vi "testRollover.vi"() -> ()   [LabVIEW 2017]
uses:
  <vilib>/addons/InsightCM/Utilities/Analysis/Vibration/controls/digital tach state.ctl
  <vilib>/addons/InsightCM/Utilities/Analysis/Vibration/controls/tach state.ctl
  <vilib>/addons/InsightCM/Devices/Shared/VibrationAnalysisLoop/controls/TachometerChanAnalysisCfg.ctl
panel:
  out "stopped":bool
  out "Instant RPM":dbl
  out "next block":dbl[](array[numeric])
  out "x/y":dbl[](array[numeric])
  out "seconds":i32
  in  "Stop":bool
  in  "Tachometer":cluster{"RPM":sgl}={"RPM"=60.0} {"RPM" scale=1.0..6000.0}
  in  "Vibration":T1(array[cluster])
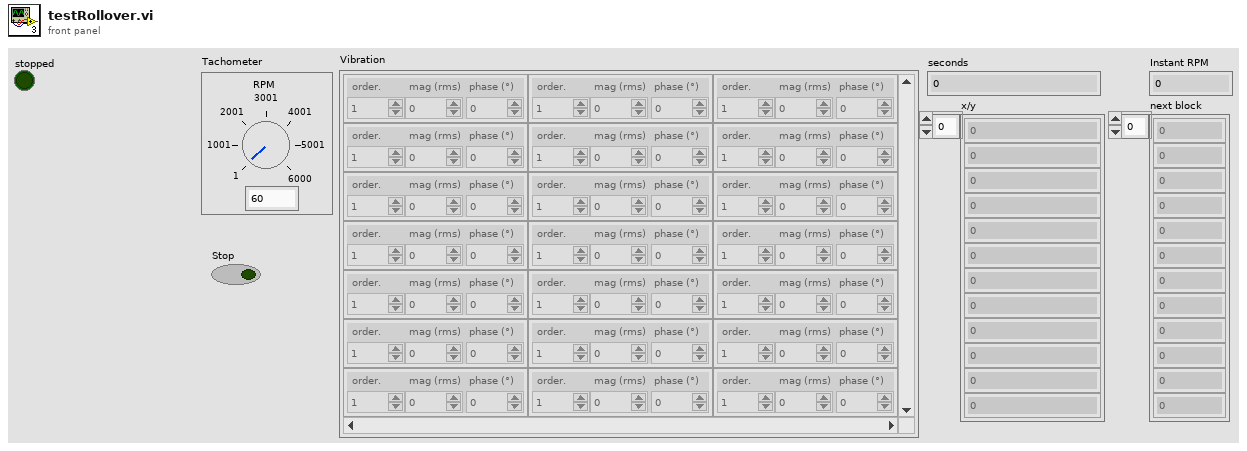
[diagram p1: front panel]
types:
  T1 = cluster{"order.":dbl, "mag (rms)":dbl, "phase (°)":dbl}[][]
  T2 = typedef "tach state.ctl" = cluster{"analog tach state":cluster{"last value":dbl, "edge state":cluster{"processed data":dbl, "buffer data":dbl[]}}, "speed state":cluster{"state":enum16{"0 Pulses", "1 Pulse", "2+ Pulses"}, "last pulse position":dbl, "RPM":dbl, "Empty Blocks":i32}, "Reset":bool, "digital tach state in":T3}
  T3 = typedef "digital tach state.ctl" = cluster{dbl[], i32, "not enough pulses?":bool, "pulse buffer out":dbl[], i32, "final state":dbl[], "duration":dbl, "reset":bool, "overflow state":cluster{"low speed state":cluster{dbl, ext}, "counter state":cluster{"counter task type":enum16{"period measurement", "event counting"}, "t":dbl, "t":dbl}}, "OS Clk Start":dbl}
  T4 = typedef "AnalysisBOP.lvlib/TachometerChanAnalysisCfg.ctl" = cluster{"Wfm Index":i32, "ChannelName":string, "ChannelID":string, "PulsesPerRevolution":sgl, "TachometerThreshold":sgl, "TachometerSlope":string, "TachometerHysteresis":sgl, "sampleRate":dbl, "tachometerType":string, "Analysis Wfm Index":i32}
  T5 = typedef "rolloverState.ctl" = cluster{"prev value":u32, "total add":dbl}
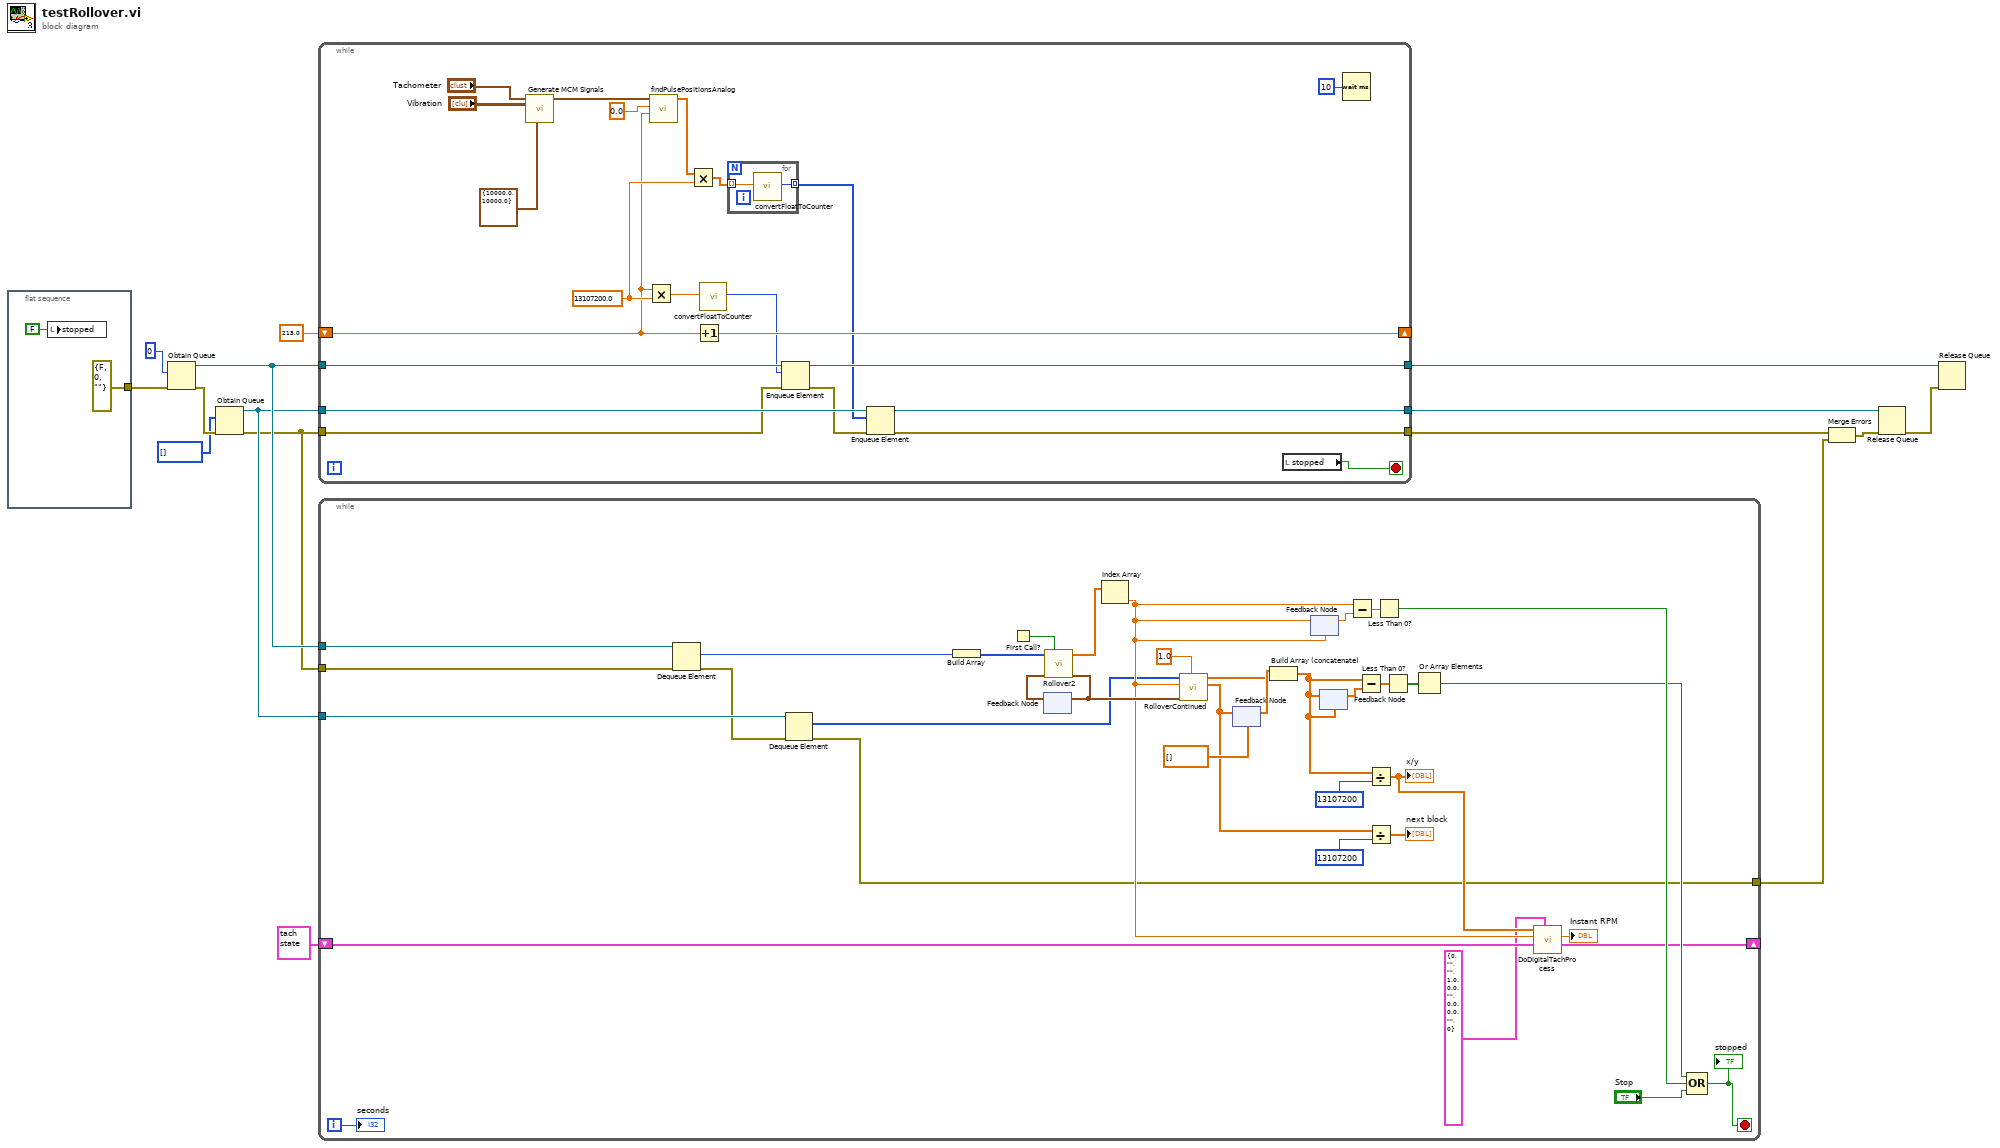
[diagram p0: block diagram]
diagram:
  n1 = flat-sequence {
    tunnel: [errorcluster {"status"=FALSE, "code"=0, "source"=""} ("error in (no error)")] -> w1
    frame #0 {
      n2 = local write "stopped"(FALSE ("stopped")) -> ()
    }
  }
  n3 = Obtain Queue(element data type=0, error in (no error)=w1) -> (queue out=w10:refnum<queue>, error out=w12:errorcluster)  [unwired: 3 in, 1 out]
  n4 = Obtain Queue(element data type=i32[] [], error in (no error)=w12) -> (queue out=w9:refnum<queue>, error out=w8:errorcluster)  [unwired: 3 in, 1 out]
  n5 = while {
    shift-right: [w29] -> _
    shift-left: 213.0 -> [w30]
    tunnel: w10 -> [w28]
    tunnel: w8 -> [w25]
    tunnel: w9 -> [w26]
    tunnel: [w23] -> w7
    tunnel: [w22] -> w5
    tunnel: [w21] -> w3
    stop <- w20 stop-if-true
    w38 = 13107200.0
    n6 = call <vilib>:"Generate MCM Signals.vi"("sampling info"=cluster{"Fs":dbl, "#s":dbl} {"Fs"=10000.0, "#s"=10000.0}, "Vibration"="Vibration", "Tachometer"="Tachometer") -> ("Tach signal"=w37:waveform(dbl))  [unwired: 6 in, 2 out]
    n7 = Multiply(x=w30, y=w38) -> (x*y=w31:dbl)
    n8 = call <vilib>:"findPulsePositionsAnalog.vi"("t0"=w30, "Level"=0.0, "Tach signal"=w37) -> ("pulse positions"=w35:dbl[])  [unwired: 8 in]
    n9 = Multiply(x=w35, y=w38) -> (x*y=w36:dbl[])
    n10 = Increment(x=w30) -> (x+1=w29:dbl)
    n11 = call <vilib>:"convertFloatToCounter.vi"("Numeric"=w31) -> ("Counter Version"=w27:u32)  [unwired: 10 in]
    n12 = for {
      tunnel: w36 -> [w41] mode=indexing
      tunnel: [w40] -> w18 mode=indexing
      n13 = call <vilib>:"convertFloatToCounter.vi"("Numeric"=w41) -> ("Counter Version"=w40:u32)  [unwired: 10 in]
    }
    n14 = Enqueue Element(queue=w28, element=w27, error in (no error)=w25) -> (queue out=w21:refnum<queue>, error out=w24:errorcluster)  [unwired: 1 in, 1 out]
    n15 = Enqueue Element(queue=w26, element=w18, error in (no error)=w24) -> (queue out=w22:refnum<queue>, error out=w23:errorcluster)  [unwired: 1 in, 1 out]
    n16 = local read "stopped"() -> (w20:bool)
    n17 = Wait (ms)(milliseconds to wait=u32 10) -> ()  [unwired: 1 out]
  }
  n18 = while {
    shift-right: [w52] -> _
    shift-left: T2 {"analog tach state"={"last value"=0.0, "edge state"={"processed data"=0.0, "buffer data"=[]}}, "speed state"={"state"=enum."0 Pulses", "last pulse position"=0.0, "RPM"=0.0, "Empty Blocks"=0}, "Reset"=FALSE, "digital tach state in"={[], 0, "not enough pulses?"=FALSE, "pulse buffer out"=[], 0, "final state"=[], "duration"=0.0, "reset"=FALSE, "overflow state"={"low speed state"={0.0, 0.0}, "counter state"={"counter task type"=enum."period measurement", "t"=0.0, "t"=0.0}}, "OS Clk Start"=0.0}} ("tach state out") -> [w51]
    tunnel: w10 -> [w48]
    tunnel: w9 -> [w46]
    tunnel: w8 -> [w43]
    tunnel: [w42] -> w6
    i -> [w68]
    stop <- w71 stop-if-true
    n19 = Dequeue Element(queue=w48, error in (no error)=w43) -> (element=w47:i32, error out=w44:errorcluster)  [unwired: 1 in, 2 out]
    n20 = Dequeue Element(queue=w46, error in (no error)=w44) -> (element=w45:i32[], error out=w42:errorcluster)  [unwired: 1 in, 2 out]
    n21 = Build Array(w47) -> (w76:i32[])
    n22 = First Call?() -> (First Call?: T/F=w78:bool)
    n23 = feedback #1() -> (w77:T5)  [unwired: 1 in]
    n24 = call <vilib>:"Rollover2.vi"("reset"=w78, "rollover state"=w77, "counter"=w76) -> ("rollover state"=w75:T5, "counter"=w74:dbl[])  [unwired: 7 in]
    n25 = feedback-in #1(w75) -> ()
    n26 = Index Array(array=w74) -> (element=w53:dbl)  [unwired: 1 in]
    n27 = call <vilib>:"RolloverContinued.vi"("acq block size (s)"=1.0, "rollover state"=w75, "OSClkStart"=w53, "counter"=w45) -> ("next block"=w56:dbl[], "this block"=w60:dbl[])  [unwired: 4 in, 2 out]
    n28 = feedback #2(dbl[] [] ("next block")) -> (w61:dbl[])
    n29 = feedback-in #2(w56) -> ()
    n30 = Build Array (concatenate)(w61, w60) -> (w59:dbl[])
    n31 = feedback-in #3(w53) -> ()
    n32 = feedback #3(w53) -> (w73:dbl)
    n33 = feedback #4(w59) -> (w66:dbl[])
    n34 = feedback-in #4(w59) -> ()
    n35 = Subtract(x=w53, y=w73) -> (x-y=w70:dbl)
    n36 = Subtract(x=w59, y=w66) -> (x-y=w67:dbl[])
    n37 = Divide(x=w59, y=13107200) -> (x/y=w54:dbl[])
    "x/y" <- w54
    n38 = Divide(x=w56, y=13107200) -> (x/y=→"next block":dbl[])
    n39 = Less Than 0?(x=w70) -> (x < 0?=w69:bool)
    n40 = Less Than 0?(x=w67) -> (x < 0?=w65:bool[])
    n41 = Or Array Elements(Boolean array=w65) -> (logical OR=w64:bool)
    n42 = call <vilib>:"DoDigitalTachProcess.vi"("TachometerChanAnalysisConfig"=T4 {"Wfm Index"=0, "ChannelName"="", "ChannelID"="", "PulsesPerRevolution"=1.0, "TachometerThreshold"=0.0, "TachometerSlope"="", "TachometerHysteresis"=0.0, "sampleRate"=0.0, "tachometerType"="", "Analysis Wfm Index"=0}, "tach state in"=w51, "OS Clk Start"=w53, "pulses"=w54) -> ("tach state out"=w52:T2, "Instant RPM"=→"Instant RPM":dbl)  [unwired: 4 in, 2 out]
    n43 = Compound Arithmetic op=OR(w64, w69, "Stop") -> (w71:bool)
    "stopped" <- w71
    "seconds" <- w68
  }
  n44 = Merge Errors(w7, w6) -> (w4:errorcluster)
  n45 = Release Queue(queue=w5, error in (no error)=w4) -> (error out=w2:errorcluster)  [unwired: 1 in, 2 out]
  n46 = Release Queue(queue=w3, error in (no error)=w2) -> ()  [unwired: 1 in, 3 out]
